vi "Test - Draw Teapot.vi"() -> ()   [LabVIEW 2022 SP3, in "Raster.lvlib"] (continued)
"y"=162.16495, "z"=0.9845819}, "UV"={"u"=0.0, "v"=0.0}, "Colour"=12517256}, "Vertex 2"={"Position"={"x"=543.45624, "y"=145.25499, "z"=0.98474205}, "UV"={"u"=0.0, "v"=0.0}, "Colour"=12517256}, "Vertex 3"={"Position"={"x"=502.52356, "y"=139.52065, "z"=0.9841747}, "UV"={"u"=0.0, "v"=0.0}, "Colour"=12517256}, "Alpha"=0.0, "Alpha Blending Enabled"=FALSE, "Colour"=5006902}, {"Vertex 1"={"Position"={"x"=354.40778, "y"=102.34398, "z"=0.9847698}, "UV"={"u"=0.0, "v"=0.0}, "Colour"=12517256}, "Vertex 2"={"Position"={"x"=351.39496, "y"=110.63302, "z"=0.984421}, "UV"={"u"=0.0, "v"=0.0}, "Colour"=12517256}, "Vertex 3"={"Position"={"x"=400.0, "y"=109.232285, "z"=0.9843054}, "UV"={"u"=0.0, "v"=0.0}, "Colour"=12517256}, "Alpha"=0.0, "Alpha Blending Enabled"=FALSE, "Colour"=395268}, {"Vertex 1"={"Position"={"x"=542.4723, "y"=251.44232, "z"=0.9847784}, "UV"={"u"=0.0, "v"=0.0}, "Colour"=12517256}, "Vertex 2"={"Position"={"x"=546.1793, "y"=227.81743, "z"=0.98464125}, "UV"={"u"=0.0, "v"=0.0}, "Colour"=12517256}, "Vertex 3"={"Position"={"x"=504.54324, "y"=225.08987, "z"=0.98405904}, "UV"={"u"=0.0, "v"=0.0}, "Colour"=12517256}, "Alpha"=0.0, "Alpha Blending Enabled"=FALSE, "Colour"=9947756}, {"Vertex 1"={"Position"={"x"=350.56738, "y"=298.80087, "z"=0.9843252}, "UV"={"u"=0.0, "v"=0.0}, "Colour"=12517256}, "Vertex 2"={"Position"={"x"=353.04034, "y"=323.3558, "z"=0.9846115}, "UV"={"u"=0.0, "v"=0.0}, "Colour"=12517256}, "Vertex 3"={"Position"={"x"=400.0, "y"=323.52267, "z"=0.9845012}, "UV"={"u"=0.0, "v"=0.0}, "Colour"=12517256}, "Alpha"=0.0, "Alpha Blending Enabled"=FALSE, "Colour"=11463036}, {"Vertex 1"={"Position"={"x"=301.7536, "y"=274.33585, "z"=0.9844198}, "UV"={"u"=0.0, "v"=0.0}, "Colour"=12517256}, "Vertex 2"={"Position"={"x"=298.20557, "y"=249.65573, "z"=0.9842166}, "UV"={"u"=0.0, "v"=0.0}, "Colour"=12517256}, "Vertex 3"={"Position"={"x"=257.52774, "y"=251.44232, "z"=0.9847784}, "UV"={"u"=0.0, "v"=0.0}, "Colour"=12517256}, "Alpha"=0.0, "Alpha Blending Enabled"=FALSE, "Colour"=10343024}, {"Vertex 1"={"Position"={"x"=301.7536, "y"=274.33585, "z"=0.9844198}, "UV"={"u"=0.0, "v"=0.0}, "Colour"=12517256}, "Vertex 2"={"Position"={"x"=305.9204, "y"=298.8263, "z"=0.9846586}, "UV"={"u"=0.0, "v"=0.0}, "Colour"=12517256}, "Vertex 3"={"Position"={"x"=350.56738, "y"=298.80087, "z"=0.9843252}, "UV"={"u"=0.0, "v"=0.0}, "Colour"=12517256}, "Alpha"=0.0, "Alpha Blending Enabled"=FALSE, "Colour"=11002232}, {"Vertex 1"={"Position"={"x"=400.0, "y"=100.973206, "z"=0.98466384}, "UV"={"u"=0.0, "v"=0.0}, "Colour"=12517256}, "Vertex 2"={"Position"={"x"=400.0, "y"=109.232285, "z"=0.9843054}, "UV"={"u"=0.0, "v"=0.0}, "Colour"=12517256}, "Vertex 3"={"Position"={"x"=448.60507, "y"=110.63302, "z"=0.984421}, "UV"={"u"=0.0, "v"=0.0}, "Colour"=12517256}, "Alpha"=0.0, "Alpha Blending Enabled"=FALSE, "Colour"=395268}, {"Vertex 1"={"Position"={"x"=497.92285, "y"=125.52894, "z"=0.98443836}, "UV"={"u"=0.0, "v"=0.0}, "Colour"=12517256}, "Vertex 2"={"Position"={"x"=502.52356, "y"=139.52065, "z"=0.9841747}, "UV"={"u"=0.0, "v"=0.0}, "Colour"=12517256}, "Vertex 3"={"Position"={"x"=543.45624, "y"=145.25499, "z"=0.98474205}, "UV"={"u"=0.0, "v"=0.0}, "Colour"=12517256}, "Alpha"=0.0, "Alpha Blending Enabled"=FALSE, "Colour"=2964512}, {"Vertex 1"={"Position"={"x"=400.0, "y"=298.79187, "z"=0.98420686}, "UV"={"u"=0.0, "v"=0.0}, "Colour"=12517256}, "Vertex 2"={"Position"={"x"=400.0, "y"=323.52267, "z"=0.9845012}, "UV"={"u"=0.0, "v"=0.0}, "Colour"=12517256}, "Vertex 3"={"Position"={"x"=446.95963, "y"=323.3558, "z"=0.9846115}, "UV"={"u"=0.0, "v"=0.0}, "Colour"=12517256}, "Alpha"=0.0, "Alpha Blending Enabled"=FALSE, "Colour"=11463036}, {"Vertex 1"={"Position"={"x"=256.5438, "y"=145.25499, "z"=0.98474205}, "UV"={"u"=0.0, "v"=0.0}, "Colour"=12517256}, "Vertex 2"={"Position"={"x"=252.2155, "y"=162.16495, "z"=0.9845819}, "UV"={"u"=0.0, "v"=0.0}, "Colour"=12517256}, "Vertex 3"={"Position"={"x"=294.26508, "y"=156.89722, "z"=0.9839907}, "UV"={"u"=0.0, "v"=0.0}, "Colour"=12517256}, "Alpha"=0.0, "Alpha Blending Enabled"=FALSE, "Colour"=5006902}, {"Vertex 1"={"Position"={"x"=307.46243, "y"=114.58211, "z"=0.98474693}, "UV"={"u"=0.0, "v"=0.0}, "Colour"=12517256}, "Vertex 2"={"Position"={"x"=302.07715, "y"=125.52894, "z"=0.98443836}, "UV"={"u"=0.0, "v"=0.0}, "Colour"=12517256}, "Vertex 3"={"Position"={"x"=348.50262, "y"=121.591866, "z"=0.98408604}, "UV"={"u"=0.0, "v"=0.0}, "Colour"=12517256}, "Alpha"=0.0, "Alpha Blending Enabled"=FALSE, "Colour"=1581073}, {"Vertex 1"={"Position"={"x"=348.50262, "y"=121.591866, "z"=0.98408604}, "UV"={"u"=0.0, "v"=0.0}, "Colour"=12517256}, "Vertex 2"={"Position"={"x"=351.39496, "y"=110.63302, "z"=0.984421}, "UV"={"u"=0.0, "v"=0.0}, "Colour"=12517256}, "Vertex 3"={"Position"={"x"=307.46243, "y"=114.58211, "z"=0.98474693}, "UV"={"u"=0.0, "v"=0.0}, "Colour"=12517256}, "Alpha"=0.0, "Alpha Blending Enabled"=FALSE, "Colour"=1581073}, {"Vertex 1"={"Position"={"x"=251.43709, "y"=204.66248, "z"=0.9845531}, "UV"={"u"=0.0, "v"=0.0}, "Colour"=12517256}, "Vertex 2"={"Position"={"x"=253.82066, "y"=227.81743, "z"=0.98464125}, "UV"={"u"=0.0, "v"=0.0}, "Colour"=12517256}, "Vertex 3"={"Position"={"x"=295.45676, "y"=225.08987, "z"=0.98405904}, "UV"={"u"=0.0, "v"=0.0}, "Colour"=12517256}, "Alpha"=0.0, "Alpha Blending Enabled"=FALSE, "Colour"=9355110}, {"Vertex 1"={"Position"={"x"=546.1793, "y"=227.81743, "z"=0.98464125}, "UV"={"u"=0.0, "v"=0.0}, "Colour"=12517256}, "Vertex 2"={"Position"={"x"=548.5629, "y"=204.66248, "z"=0.9845531}, "UV"={"u"=0.0, "v"=0.0}, "Colour"=12517256}, "Vertex 3"={"Position"={"x"=506.31323, "y"=200.99902, "z"=0.98395765}, "UV"={"u"=0.0, "v"=0.0}, "Colour"=12517256}, "Alpha"=0.0, "Alpha Blending Enabled"=FALSE, "Colour"=9355110}, {"Vertex 1"={"Position"={"x"=494.0796, "y"=298.8263, "z"=0.9846586}, "UV"={"u"=0.0, "v"=0.0}, "Colour"=12517256}, "Vertex 2"={"Position"={"x"=498.2464, "y"=274.33585, "z"=0.9844198}, "UV"={"u"=0.0, "v"=0.0}, "Colour"=12517256}, "Vertex 3"={"Position"={"x"=451.6715, "y"=273.75476, "z"=0.9840659}, "UV"={"u"=0.0, "v"=0.0}, "Colour"=12517256}, "Alpha"=0.0, "Alpha Blending Enabled"=FALSE, "Colour"=11002232}, {"Vertex 1"={"Position"={"x"=446.95963, "y"=323.3558, "z"=0.9846115}, "UV"={"u"=0.0, "v"=0.0}, "Colour"=12517256}, "Vertex 2"={"Position"={"x"=449.43246, "y"=298.80087, "z"=0.9843252}, "UV"={"u"=0.0, "v"=0.0}, "Colour"=12517256}, "Vertex 3"={"Position"={"x"=400.0, "y"=298.79187, "z"=0.98420686}, "UV"={"u"=0.0, "v"=0.0}, "Colour"=12517256}, "Alpha"=0.0, "Alpha Blending Enabled"=FALSE, "Colour"=11463036}, {"Vertex 1"={"Position"={"x"=549.402, "y"=182.33759, "z"=0.9845221}, "UV"={"u"=0.0, "v"=0.0}, "Colour"=12517256}, "Vertex 2"={"Position"={"x"=547.78455, "y"=162.16495, "z"=0.9845819}, "UV"={"u"=0.0, "v"=0.0}, "Colour"=12517256}, "Vertex 3"={"Position"={"x"=505.73492, "y"=156.89722, "z"=0.9839907}, "UV"={"u"=0.0, "v"=0.0}, "Colour"=12517256}, "Alpha"=0.0, "Alpha Blending Enabled"=FALSE, "Colour"=7180878}, {"Vertex 1"={"Position"={"x"=504.54324, "y"=225.08987, "z"=0.98405904}, "UV"={"u"=0.0, "v"=0.0}, "Colour"=12517256}, "Vertex 2"={"Position"={"x"=501.79443, "y"=249.65573, "z"=0.9842166}, "UV"={"u"=0.0, "v"=0.0}, "Colour"=12517256}, "Vertex 3"={"Position"={"x"=542.4723, "y"=251.44232, "z"=0.9847784}, "UV"={"u"=0.0, "v"=0.0}, "Colour"=12517256}, "Alpha"=0.0, "Alpha Blending Enabled"=FALSE, "Colour"=9947756}, {"Vertex 1"={"Position"={"x"=451.6715, "y"=273.75476, "z"=0.9840659}, "UV"={"u"=0.0, "v"=0.0}, "Colour"=12517256}, "Vertex 2"={"Position"={"x"=449.43246, "y"=298.80087, "z"=0.9843252}, "UV"={"u"=0.0, "v"=0.0}, "Colour"=12517256}, "Vertex 3"={"Position"={"x"=494.0796, "y"=298.8263, "z"=0.9846586}, "UV"={"u"=0.0, "v"=0.0}, "Colour"=12517256}, "Alpha"=0.0, "Alpha Blending Enabled"=FALSE, "Colour"=11002232}, {"Vertex 1"={"Position"={"x"=400.0, "y"=323.52267, "z"=0.9845012}, "UV"={"u"=0.0, "v"=0.0}, "Colour"=12517256}, "Vertex 2"={"Position"={"x"=400.0, "y"=298.79187, "z"=0.98420686}, "UV"={"u"=0.0, "v"=0.0}, "Colour"=12517256}, "Vertex 3"={"Position"={"x"=350.56738, "y"=298.80087, "z"=0.9843252}, "UV"={"u"=0.0, "v"=0.0}, "Colour"=12517256}, "Alpha"=0.0, "Alpha Blending Enabled"=FALSE, "Colour"=11463036}, {"Vertex 1"={"Position"={"x"=250.598, "y"=182.33759, "z"=0.9845221}, "UV"={"u"=0.0, "v"=0.0}, "Colour"=12517256}, "Vertex 2"={"Position"={"x"=251.43709, "y"=204.66248, "z"=0.9845531}, "UV"={"u"=0.0, "v"=0.0}, "Colour"=12517256}, "Vertex 3"={"Position"={"x"=293.68674, "y"=200.99902, "z"=0.98395765}, "UV"={"u"=0.0, "v"=0.0}, "Colour"=12517256}, "Alpha"=0.0, "Alpha Blending Enabled"=FALSE, "Colour"=8630366}, {"Vertex 1"={"Position"={"x"=252.2155, "y"=162.16495, "z"=0.9845819}, "UV"={"u"=0.0, "v"=0.0}, "Colour"=12517256}, "Vertex 2"={"Position"={"x"=250.598, "y"=182.33759, "z"=0.9845221}, "UV"={"u"=0.0, "v"=0.0}, "Colour"=12517256}, "Vertex 3"={"Position"={"x"=293.06296, "y"=177.78967, "z"=0.9839219}, "UV"={"u"=0.0, "v"=0.0}, "Colour"=12517256}, "Alpha"=0.0, "Alpha Blending Enabled"=FALSE, "Colour"=7180878}, {"Vertex 1"={"Position"={"x"=548.5629, "y"=204.66248, "z"=0.9845531}, "UV"={"u"=0.0, "v"=0.0}, "Colour"=12517256}, "Vertex 2"={"Position"={"x"=549.402, "y"=182.33759, "z"=0.9845221}, "UV"={"u"=0.0, "v"=0.0}, "Colour"=12517256}, "Vertex 3"={"Position"={"x"=506.937, "y"=177.78967, "z"=0.9839219}, "UV"={"u"=0.0, "v"=0.0}, "Colour"=12517256}, "Alpha"=0.0, "Alpha Blending Enabled"=FALSE, "Colour"=8630366}, {"Vertex 1"={"Position"={"x"=448.60507, "y"=110.63302, "z"=0.984421}, "UV"={"u"=0.0, "v"=0.0}, "Colour"=12517256}, "Vertex 2"={"Position"={"x"=451.49738, "y"=121.591866, "z"=0.98408604}, "UV"={"u"=0.0, "v"=0.0}, "Colour"=12517256}, "Vertex 3"={"Position"={"x"=497.92285, "y"=125.52894, "z"=0.98443836}, "UV"={"u"=0.0, "v"=0.0}, "Colour"=12517256}, "Alpha"=0.0, "Alpha Blending Enabled"=FALSE, "Colour"=1581073}, {"Vertex 1"={"Position"={"x"=298.20557, "y"=249.65573, "z"=0.9842166}, "UV"={"u"=0.0, "v"=0.0}, "Colour"=12517256}, "Vertex 2"={"Position"={"x"=295.45676, "y"=225.08987, "z"=0.98405904}, "UV"={"u"=0.0, "v"=0.0}, "Colour"=12517256}, "Vertex 3"={"Position"={"x"=253.82066, "y"=227.81743, "z"=0.98464125}, "UV"={"u"=0.0, "v"=0.0}, "Colour"=12517256}, "Alpha"=0.0, "Alpha Blending Enabled"=FALSE, "Colour"=9947756}, {"Vertex 1"={"Position"={"x"=294.26508, "y"=156.89722, "z"=0.9839907}, "UV"={"u"=0.0, "v"=0.0}, "Colour"=12517256}, "Vertex 2"={"Position"={"x"=297.47644, "y"=139.52065, "z"=0.9841747}, "UV"={"u"=0.0, "v"=0.0}, "Colour"=12517256}, "Vertex 3"={"Position"={"x"=256.5438, "y"=145.25499, "z"=0.98474205}, "UV"={"u"=0.0, "v"=0.0}, "Colour"=12517256}, "Alpha"=0.0, "Alpha Blending Enabled"=FALSE, "Colour"=5006902}, {"Vertex 1"={"Position"={"x"=451.49738, "y"=121.591866, "z"=0.98408604}, "UV"={"u"=0.0, "v"=0.0}, "Colour"=12517256}, "Vertex 2"={"Position"={"x"=448.60507, "y"=110.63302, "z"=0.984421}, "UV"={"u"=0.0, "v"=0.0}, "Colour"=12517256}, "Vertex 3"={"Position"={"x"=400.0, "y"=109.232285, "z"=0.9843054}, "UV"={"u"=0.0, "v"=0.0}, "Colour"=12517256}, "Alpha"=0.0, "Alpha Blending Enabled"=FALSE, "Colour"=1778707}, {"Vertex 1"={"Position"={"x"=350.56738, "y"=298.80087, "z"=0.9843252}, "UV"={"u"=0.0, "v"=0.0}, "Colour"=12517256}, "Vertex 2"={"Position"={"x"=348.32846, "y"=273.75476, "z"=0.9840659}, "UV"={"u"=0.0, "v"=0.0}, "Colour"=12517256}, "Vertex 3"={"Position"={"x"=301.7536, "y"=274.33585, "z"=0.9844198}, "UV"={"u"=0.0, "v"=0.0}, "Colour"=12517256}, "Alpha"=0.0, "Alpha Blending Enabled"=FALSE, "Colour"=11002232}, {"Vertex 1"={"Position"={"x"=502.52356, "y"=139.52065, "z"=0.9841747}, "UV"={"u"=0.0, "v"=0.0}, "Colour"=12517256}, "Vertex 2"={"Position"={"x"=505.73492, "y"=156.89722, "z"=0.9839907}, "UV"={"u"=0.0, "v"=0.0}, "Colour"=12517256}, "Vertex 3"={"Position"={"x"=547.78455, "y"=162.16495, "z"=0.9845819}, "UV"={"u"=0.0, "v"=0.0}, "Colour"=12517256}, "Alpha"=0.0, "Alpha Blending Enabled"=FALSE, "Colour"=5006902}, {"Vertex 1"={"Position"={"x"=298.20557, "y"=249.65573, "z"=0.9842166}, "UV"={"u"=0.0, "v"=0.0}, "Colour"=12517256}, "Vertex 2"={"Position"={"x"=301.7536, "y"=274.33585, "z"=0.9844198}, "UV"={"u"=0.0, "v"=0.0}, "Colour"=12517256}, "Vertex 3"={"Position"={"x"=348.32846, "y"=273.75476, "z"=0.9840659}, "UV"={"u"=0.0, "v"=0.0}, "Colour"=12517256}, "Alpha"=0.0, "Alpha Blending Enabled"=FALSE, "Colour"=10738549}, {"Vertex 1"={"Position"={"x"=502.52356, "y"=139.52065, "z"=0.9841747}, "UV"={"u"=0.0, "v"=0.0}, "Colour"=12517256}, "Vertex 2"={"Position"={"x"=497.92285, "y"=125.52894, "z"=0.98443836}, "UV"={"u"=0.0, "v"=0.0}, "Colour"=12517256}, "Vertex 3"={"Position"={"x"=451.49738, "y"=121.591866, "z"=0.98408604}, "UV"={"u"=0.0, "v"=0.0}, "Colour"=12517256}, "Alpha"=0.0, "Alpha Blending Enabled"=FALSE, "Colour"=3294244}, {"Vertex 1"={"Position"={"x"=400.0, "y"=120.19295, "z"=0.98396087}, "UV"={"u"=0.0, "v"=0.0}, "Colour"=12517256}, "Vertex 2"={"Position"={"x"=400.0, "y"=109.232285, "z"=0.9843054}, "UV"={"u"=0.0, "v"=0.0}, "Colour"=12517256}, "Vertex 3"={"Position"={"x"=351.39496, "y"=110.63302, "z"=0.984421}, "UV"={"u"=0.0, "v"=0.0}, "Colour"=12517256}, "Alpha"=0.0, "Alpha Blending Enabled"=FALSE, "Colour"=1778707}, {"Vertex 1"={"Position"={"x"=506.31323, "y"=200.99902, "z"=0.98395765}, "UV"={"u"=0.0, "v"=0.0}, "Colour"=12517256}, "Vertex 2"={"Position"={"x"=504.54324, "y"=225.08987, "z"=0.98405904}, "UV"={"u"=0.0, "v"=0.0}, "Colour"=12517256}, "Vertex 3"={"Position"={"x"=546.1793, "y"=227.81743, "z"=0.98464125}, "UV"={"u"=0.0, "v"=0.0}, "Colour"=12517256}, "Alpha"=0.0, "Alpha Blending Enabled"=FALSE, "Colour"=9355110}, {"Vertex 1"={"Position"={"x"=348.32846, "y"=273.75476, "z"=0.9840659}, "UV"={"u"=0.0, "v"=0.0}, "Colour"=12517256}, "Vertex 2"={"Position"={"x"=350.56738, "y"=298.80087, "z"=0.9843252}, "UV"={"u"=0.0, "v"=0.0}, "Colour"=12517256}, "Vertex 3"={"Position"={"x"=400.0, "y"=298.79187, "z"=0.98420686}, "UV"={"u"=0.0, "v"=0.0}, "Colour"=12517256}, "Alpha"=0.0, "Alpha Blending Enabled"=FALSE, "Colour"=11199866}, {"Vertex 1"={"Position"={"x"=295.45676, "y"=225.08987, "z"=0.98405904}, "UV"={"u"=0.0, "v"=0.0}, "Colour"=12517256}, "Vertex 2"={"Position"={"x"=293.68674, "y"=200.99902, "z"=0.98395765}, "UV"={"u"=0.0, "v"=0.0}, "Colour"=12517256}, "Vertex 3"={"Position"={"x"=251.43709, "y"=204.66248, "z"=0.9845531}, "UV"={"u"=0.0, "v"=0.0}, "Colour"=12517256}, "Alpha"=0.0, "Alpha Blending Enabled"=FALSE, "Colour"=9355110}, {"Vertex 1"={"Position"={"x"=293.06296, "y"=177.78967, "z"=0.9839219}, "UV"={"u"=0.0, "v"=0.0}, "Colour"=12517256}, "Vertex 2"={"Position"={"x"=294.26508, "y"=156.89722, "z"=0.9839907}, "UV"={"u"=0.0, "v"=0.0}, "Colour"=12517256}, "Vertex 3"={"Position"={"x"=252.2155, "y"=162.16495, "z"=0.9845819}, "UV"={"u"=0.0, "v"=0.0}, "Colour"=12517256}, "Alpha"=0.0, "Alpha Blending Enabled"=FALSE, "Colour"=7180878}, {"Vertex 1"={"Position"={"x"=498.2464, "y"=274.33585, "z"=0.9844198}, "UV"={"u"=0.0, "v"=0.0}, "Colour"=12517256}, "Vertex 2"={"Position"={"x"=501.79443, "y"=249.65573, "z"=0.9842166}, "UV"={"u"=0.0, "v"=0.0}, "Colour"=12517256}, "Vertex 3"={"Position"={"x"=453.58133, "y"=248.47368, "z"=0.98384476}, "UV"={"u"=0.0, "v"=0.0}, "Colour"=12517256}, "Alpha"=0.0, "Alpha Blending Enabled"=FALSE, "Colour"=10738549}, {"Vertex 1"={"Position"={"x"=400.0, "y"=273.54828, "z"=0.9839401}, "UV"={"u"=0.0, "v"=0.0}, "Colour"=12517256}, "Vertex 2"={"Position"={"x"=400.0, "y"=298.79187, "z"=0.98420686}, "UV"={"u"=0.0, "v"=0.0}, "Colour"=12517256}, "Vertex 3"={"Position"={"x"=449.43246, "y"=298.80087, "z"=0.9843252}, "UV"={"u"=0.0, "v"=0.0}, "Colour"=12517256}, "Alpha"=0.0, "Alpha Blending Enabled"=FALSE, "Colour"=11199866}, {"Vertex 1"={"Position"={"x"=351.39496, "y"=110.63302, "z"=0.984421}, "UV"={"u"=0.0, "v"=0.0}, "Colour"=12517256}, "Vertex 2"={"Position"={"x"=348.50262, "y"=121.591866, "z"=0.98408604}, "UV"={"u"=0.0, "v"=0.0}, "Colour"=12517256}, "Vertex 3"={"Position"={"x"=400.0, "y"=120.19295, "z"=0.98396087}, "UV"={"u"=0.0, "v"=0.0}, "Colour"=12517256}, "Alpha"=0.0, "Alpha Blending Enabled"=FALSE, "Colour"=1778707}, {"Vertex 1"={"Position"={"x"=505.73492, "y"=156.89722, "z"=0.9839907}, "UV"={"u"=0.0, "v"=0.0}, "Colour"=12517256}, "Vertex 2"={"Position"={"x"=506.937, "y"=177.78967, "z"=0.9839219}, "UV"={"u"=0.0, "v"=0.0}, "Colour"=12517256}, "Vertex 3"={"Position"={"x"=549.402, "y"=182.33759, "z"=0.9845221}, "UV"={"u"=0.0, "v"=0.0}, "Colour"=12517256}, "Alpha"=0.0, "Alpha Blending Enabled"=FALSE, "Colour"=7180878}, {"Vertex 1"={"Position"={"x"=506.937, "y"=177.78967, "z"=0.9839219}, "UV"={"u"=0.0, "v"=0.0}, "Colour"=12517256}, "Vertex 2"={"Position"={"x"=506.31323, "y"=200.99902, "z"=0.98395765}, "UV"={"u"=0.0, "v"=0.0}, "Colour"=12517256}, "Vertex 3"={"Position"={"x"=548.5629, "y"=204.66248, "z"=0.9845531}, "UV"={"u"=0.0, "v"=0.0}, "Colour"=12517256}, "Alpha"=0.0, "Alpha Blending Enabled"=FALSE, "Colour"=8630366}, {"Vertex 1"={"Position"={"x"=302.07715, "y"=125.52894, "z"=0.98443836}, "UV"={"u"=0.0, "v"=0.0}, "Colour"=12517256}, "Vertex 2"={"Position"={"x"=297.47644, "y"=139.52065, "z"=0.9841747}, "UV"={"u"=0.0, "v"=0.0}, "Colour"=12517256}, "Vertex 3"={"Position"={"x"=346.02576, "y"=135.72502, "z"=0.9837993}, "UV"={"u"=0.0, "v"=0.0}, "Colour"=12517256}, "Alpha"=0.0, "Alpha Blending Enabled"=FALSE, "Colour"=3294244}, {"Vertex 1"={"Position"={"x"=293.68674, "y"=200.99902, "z"=0.98395765}, "UV"={"u"=0.0, "v"=0.0}, "Colour"=12517256}, "Vertex 2"={"Position"={"x"=293.06296, "y"=177.78967, "z"=0.9839219}, "UV"={"u"=0.0, "v"=0.0}, "Colour"=12517256}, "Vertex 3"={"Position"={"x"=250.598, "y"=182.33759, "z"=0.9845221}, "UV"={"u"=0.0, "v"=0.0}, "Colour"=12517256}, "Alpha"=0.0, "Alpha Blending Enabled"=FALSE, "Colour"=8630366}, {"Vertex 1"={"Position"={"x"=400.0, "y"=109.232285, "z"=0.9843054}, "UV"={"u"=0.0, "v"=0.0}, "Colour"=12517256}, "Vertex 2"={"Position"={"x"=400.0, "y"=120.19295, "z"=0.98396087}, "UV"={"u"=0.0, "v"=0.0}, "Colour"=12517256}, "Vertex 3"={"Position"={"x"=451.49738, "y"=121.591866, "z"=0.98408604}, "UV"={"u"=0.0, "v"=0.0}, "Colour"=12517256}, "Alpha"=0.0, "Alpha Blending Enabled"=FALSE, "Colour"=1778707}, {"Vertex 1"={"Position"={"x"=449.43246, "y"=298.80087, "z"=0.9843252}, "UV"={"u"=0.0, "v"=0.0}, "Colour"=12517256}, "Vertex 2"={"Position"={"x"=451.6715, "y"=273.75476, "z"=0.9840659}, "UV"={"u"=0.0, "v"=0.0}, "Colour"=12517256}, "Vertex 3"={"Position"={"x"=400.0, "y"=273.54828, "z"=0.9839401}, "UV"={"u"=0.0, "v"=0.0}, "Colour"=12517256}, "Alpha"=0.0, "Alpha Blending Enabled"=FALSE, "Colour"=11199866}, {"Vertex 1"={"Position"={"x"=453.58133, "y"=248.47368, "z"=0.98384476}, "UV"={"u"=0.0, "v"=0.0}, "Colour"=12517256}, "Vertex 2"={"Position"={"x"=451.6715, "y"=273.75476, "z"=0.9840659}, "UV"={"u"=0.0, "v"=0.0}, "Colour"=12517256}, "Vertex 3"={"Position"={"x"=498.2464, "y"=274.33585, "z"=0.9844198}, "UV"={"u"=0.0, "v"=0.0}, "Colour"=12517256}, "Alpha"=0.0, "Alpha Blending Enabled"=FALSE, "Colour"=10738549}, {"Vertex 1"={"Position"={"x"=346.02576, "y"=135.72502, "z"=0.9837993}, "UV"={"u"=0.0, "v"=0.0}, "Colour"=12517256}, "Vertex 2"={"Position"={"x"=348.50262, "y"=121.591866, "z"=0.98408604}, "UV"={"u"=0.0, "v"=0.0}, "Colour"=12517256}, "Vertex 3"={"Position"={"x"=302.07715, "y"=125.52894, "z"=0.98443836}, "UV"={"u"=0.0, "v"=0.0}, "Colour"=12517256}, "Alpha"=0.0, "Alpha Blending Enabled"=FALSE, "Colour"=3294244}, {"Vertex 1"={"Position"={"x"=400.0, "y"=298.79187, "z"=0.98420686}, "UV"={"u"=0.0, "v"=0.0}, "Colour"=12517256}, "Vertex 2"={"Position"={"x"=400.0, "y"=273.54828, "z"=0.9839401}, "UV"={"u"=0.0, "v"=0.0}, "Colour"=12517256}, "Vertex 3"={"Position"={"x"=348.32846, "y"=273.75476, "z"=0.9840659}, "UV"={"u"=0.0, "v"=0.0}, "Colour"=12517256}, "Alpha"=0.0, "Alpha Blending Enabled"=FALSE, "Colour"=11199866}, {"Vertex 1"={"Position"={"x"=348.32846, "y"=273.75476, "z"=0.9840659}, "UV"={"u"=0.0, "v"=0.0}, "Colour"=12517256}, "Vertex 2"={"Position"={"x"=346.41867, "y"=248.47368, "z"=0.98384476}, "UV"={"u"=0.0, "v"=0.0}, "Colour"=12517256}, "Vertex 3"={"Position"={"x"=298.20557, "y"=249.65573, "z"=0.9842166}, "UV"={"u"=0.0, "v"=0.0}, "Colour"=12517256}, "Alpha"=0.0, "Alpha Blending Enabled"=FALSE, "Colour"=10738549}, {"Vertex 1"={"Position"={"x"=295.45676, "y"=225.08987, "z"=0.98405904}, "UV"={"u"=0.0, "v"=0.0}, "Colour"=12517256}, "Vertex 2"={"Position"={"x"=298.20557, "y"=249.65573, "z"=0.9842166}, "UV"={"u"=0.0, "v"=0.0}, "Colour"=12517256}, "Vertex 3"={"Position"={"x"=346.41867, "y"=248.47368, "z"=0.98384476}, "UV"={"u"=0.0, "v"=0.0}, "Colour"=12517256}, "Alpha"=0.0, "Alpha Blending Enabled"=FALSE, "Colour"=10343280}, {"Vertex 1"={"Position"={"x"=451.49738, "y"=121.591866, "z"=0.98408604}, "UV"={"u"=0.0, "v"=0.0}, "Colour"=12517256}, "Vertex 2"={"Position"={"x"=453.97424, "y"=135.72502, "z"=0.9837993}, "UV"={"u"=0.0, "v"=0.0}, "Colour"=12517256}, "Vertex 3"={"Position"={"x"=502.52356, "y"=139.52065, "z"=0.9841747}, "UV"={"u"=0.0, "v"=0.0}, "Colour"=12517256}, "Alpha"=0.0, "Alpha Blending Enabled"=FALSE, "Colour"=3294244}, {"Vertex 1"={"Position"={"x"=505.73492, "y"=156.89722, "z"=0.9839907}, "UV"={"u"=0.0, "v"=0.0}, "Colour"=12517256}, "Vertex 2"={"Position"={"x"=502.52356, "y"=139.52065, "z"=0.9841747}, "UV"={"u"=0.0, "v"=0.0}, "Colour"=12517256}, "Vertex 3"={"Position"={"x"=453.97424, "y"=135.72502, "z"=0.9837993}, "UV"={"u"=0.0, "v"=0.0}, "Colour"=12517256}, "Alpha"=0.0, "Alpha Blending Enabled"=FALSE, "Colour"=5402171}, {"Vertex 1"={"Position"={"x"=501.79443, "y"=249.65573, "z"=0.9842166}, "UV"={"u"=0.0, "v"=0.0}, "Colour"=12517256}, "Vertex 2"={"Position"={"x"=504.54324, "y"=225.08987, "z"=0.98405904}, "UV"={"u"=0.0, "v"=0.0}, "Colour"=12517256}, "Vertex 3"={"Position"={"x"=455.0632, "y"=223.28236, "z"=0.9836732}, "UV"={"u"=0.0, "v"=0.0}, "Colour"=12517256}, "Alpha"=0.0, "Alpha Blending Enabled"=FALSE, "Colour"=10343280}, {"Vertex 1"={"Position"={"x"=346.41867, "y"=248.47368, "z"=0.98384476}, "UV"={"u"=0.0, "v"=0.0}, "Colour"=12517256}, "Vertex 2"={"Position"={"x"=348.32846, "y"=273.75476, "z"=0.9840659}, "UV"={"u"=0.0, "v"=0.0}, "Colour"=12517256}, "Vertex 3"={"Position"={"x"=400.0, "y"=273.54828, "z"=0.9839401}, "UV"={"u"=0.0, "v"=0.0}, "Colour"=12517256}, "Alpha"=0.0, "Alpha Blending Enabled"=FALSE, "Colour"=10936183}, {"Vertex 1"={"Position"={"x"=453.97424, "y"=135.72502, "z"=0.9837993}, "UV"={"u"=0.0, "v"=0.0}, "Colour"=12517256}, "Vertex 2"={"Position"={"x"=451.49738, "y"=121.591866, "z"=0.98408604}, "UV"={"u"=0.0, "v"=0.0}, "Colour"=12517256}, "Vertex 3"={"Position"={"x"=400.0, "y"=120.19295, "z"=0.98396087}, "UV"={"u"=0.0, "v"=0.0}, "Colour"=12517256}, "Alpha"=0.0, "Alpha Blending Enabled"=FALSE, "Colour"=3491878}, {"Vertex 1"={"Position"={"x"=297.47644, "y"=139.52065, "z"=0.9841747}, "UV"={"u"=0.0, "v"=0.0}, "Colour"=12517256}, "Vertex 2"={"Position"={"x"=294.26508, "y"=156.89722, "z"=0.9839907}, "UV"={"u"=0.0, "v"=0.0}, "Colour"=12517256}, "Vertex 3"={"Position"={"x"=344.29382, "y"=153.40399, "z"=0.9835987}, "UV"={"u"=0.0, "v"=0.0}, "Colour"=12517256}, "Alpha"=0.0, "Alpha Blending Enabled"=FALSE, "Colour"=5402171}, {"Vertex 1"={"Position"={"x"=455.0632, "y"=223.28236, "z"=0.9836732}, "UV"={"u"=0.0, "v"=0.0}, "Colour"=12517256}, "Vertex 2"={"Position"={"x"=453.58133, "y"=248.47368, "z"=0.98384476}, "UV"={"u"=0.0, "v"=0.0}, "Colour"=12517256}, "Vertex 3"={"Position"={"x"=501.79443, "y"=249.65573, "z"=0.9842166}, "UV"={"u"=0.0, "v"=0.0}, "Colour"=12517256}, "Alpha"=0.0, "Alpha Blending Enabled"=FALSE, "Colour"=10343280}, {"Vertex 1"={"Position"={"x"=400.0, "y"=248.05318, "z"=0.98371255}, "UV"={"u"=0.0, "v"=0.0}, "Colour"=12517256}, "Vertex 2"={"Position"={"x"=400.0, "y"=273.54828, "z"=0.9839401}, "UV"={"u"=0.0, "v"=0.0}, "Colour"=12517256}, "Vertex 3"={"Position"={"x"=451.6715, "y"=273.75476, "z"=0.9840659}, "UV"={"u"=0.0, "v"=0.0}, "Colour"=12517256}, "Alpha"=0.0, "Alpha Blending Enabled"=FALSE, "Colour"=10936183}, {"Vertex 1"={"Position"={"x"=400.0, "y"=134.37457, "z"=0.9836657}, "UV"={"u"=0.0, "v"=0.0}, "Colour"=12517256}, "Vertex 2"={"Position"={"x"=400.0, "y"=120.19295, "z"=0.98396087}, "UV"={"u"=0.0, "v"=0.0}, "Colour"=12517256}, "Vertex 3"={"Position"={"x"=348.50262, "y"=121.591866, "z"=0.98408604}, "UV"={"u"=0.0, "v"=0.0}, "Colour"=12517256}, "Alpha"=0.0, "Alpha Blending Enabled"=FALSE, "Colour"=3491878}, {"Vertex 1"={"Position"={"x"=293.68674, "y"=200.99902, "z"=0.98395765}, "UV"={"u"=0.0, "v"=0.0}, "Colour"=12517256}, "Vertex 2"={"Position"={"x"=295.45676, "y"=225.08987, "z"=0.98405904}, "UV"={"u"=0.0, "v"=0.0}, "Colour"=12517256}, "Vertex 3"={"Position"={"x"=344.93683, "y"=223.28236, "z"=0.9836732}, "UV"={"u"=0.0, "v"=0.0}, "Colour"=12517256}, "Alpha"=0.0, "Alpha Blending Enabled"=FALSE, "Colour"=9816170}, {"Vertex 1"={"Position"={"x"=451.6715, "y"=273.75476, "z"=0.9840659}, "UV"={"u"=0.0, "v"=0.0}, "Colour"=12517256}, "Vertex 2"={"Position"={"x"=453.58133, "y"=248.47368, "z"=0.98384476}, "UV"={"u"=0.0, "v"=0.0}, "Colour"=12517256}, "Vertex 3"={"Position"={"x"=400.0, "y"=248.05318, "z"=0.98371255}, "UV"={"u"=0.0, "v"=0.0}, "Colour"=12517256}, "Alpha"=0.0, "Alpha Blending Enabled"=FALSE, "Colour"=10936183}, {"Vertex 1"={"Position"={"x"=504.54324, "y"=225.08987, "z"=0.98405904}, "UV"={"u"=0.0, "v"=0.0}, "Colour"=12517256}, "Vertex 2"={"Position"={"x"=506.31323, "y"=200.99902, "z"=0.98395765}, "UV"={"u"=0.0, "v"=0.0}, "Colour"=12517256}, "Vertex 3"={"Position"={"x"=456.01822, "y"=198.56883, "z"=0.9835626}, "UV"={"u"=0.0, "v"=0.0}, "Colour"=12517256}, "Alpha"=0.0, "Alpha Blending Enabled"=FALSE, "Colour"=9816170}, {"Vertex 1"={"Position"={"x"=346.41867, "y"=248.47368, "z"=0.98384476}, "UV"={"u"=0.0, "v"=0.0}, "Colour"=12517256}, "Vertex 2"={"Position"={"x"=344.93683, "y"=223.28236, "z"=0.9836732}, "UV"={"u"=0.0, "v"=0.0}, "Colour"=12517256}, "Vertex 3"={"Position"={"x"=295.45676, "y"=225.08987, "z"=0.98405904}, "UV"={"u"=0.0, "v"=0.0}, "Colour"=12517256}, "Alpha"=0.0, "Alpha Blending Enabled"=FALSE, "Colour"=10343280}, {"Vertex 1"={"Position"={"x"=344.29382, "y"=153.40399, "z"=0.9835987}, "UV"={"u"=0.0, "v"=0.0}, "Colour"=12517256}, "Vertex 2"={"Position"={"x"=346.02576, "y"=135.72502, "z"=0.9837993}, "UV"={"u"=0.0, "v"=0.0}, "Colour"=12517256}, "Vertex 3"={"Position"={"x"=297.47644, "y"=139.52065, "z"=0.9841747}, "UV"={"u"=0.0, "v"=0.0}, "Colour"=12517256}, "Alpha"=0.0, "Alpha Blending Enabled"=FALSE, "Colour"=5402171}, {"Vertex 1"={"Position"={"x"=348.50262, "y"=121.591866, "z"=0.98408604}, "UV"={"u"=0.0, "v"=0.0}, "Colour"=12517256}, "Vertex 2"={"Position"={"x"=346.02576, "y"=135.72502, "z"=0.9837993}, "UV"={"u"=0.0, "v"=0.0}, "Colour"=12517256}, "Vertex 3"={"Position"={"x"=400.0, "y"=134.37457, "z"=0.9836657}, "UV"={"u"=0.0, "v"=0.0}, "Colour"=12517256}, "Alpha"=0.0, "Alpha Blending Enabled"=FALSE, "Colour"=3491878}, {"Vertex 1"={"Position"={"x"=506.937, "y"=177.78967, "z"=0.9839219}, "UV"={"u"=0.0, "v"=0.0}, "Colour"=12517256}, "Vertex 2"={"Position"={"x"=505.73492, "y"=156.89722, "z"=0.9839907}, "UV"={"u"=0.0, "v"=0.0}, "Colour"=12517256}, "Vertex 3"={"Position"={"x"=455.7062, "y"=153.40399, "z"=0.9835987}, "UV"={"u"=0.0, "v"=0.0}, "Colour"=12517256}, "Alpha"=0.0, "Alpha Blending Enabled"=FALSE, "Colour"=7576403}, {"Vertex 1"={"Position"={"x"=400.0, "y"=273.54828, "z"=0.9839401}, "UV"={"u"=0.0, "v"=0.0}, "Colour"=12517256}, "Vertex 2"={"Position"={"x"=400.0, "y"=248.05318, "z"=0.98371255}, "UV"={"u"=0.0, "v"=0.0}, "Colour"=12517256}, "Vertex 3"={"Position"={"x"=346.41867, "y"=248.47368, "z"=0.98384476}, "UV"={"u"=0.0, "v"=0.0}, "Colour"=12517256}, "Alpha"=0.0, "Alpha Blending Enabled"=FALSE, "Colour"=10936183}, {"Vertex 1"={"Position"={"x"=293.06296, "y"=177.78967, "z"=0.9839219}, "UV"={"u"=0.0, "v"=0.0}, "Colour"=12517256}, "Vertex 2"={"Position"={"x"=293.68674, "y"=200.99902, "z"=0.98395765}, "UV"={"u"=0.0, "v"=0.0}, "Colour"=12517256}, "Vertex 3"={"Position"={"x"=343.98178, "y"=198.56883, "z"=0.9835626}, "UV"={"u"=0.0, "v"=0.0}, "Colour"=12517256}, "Alpha"=0.0, "Alpha Blending Enabled"=FALSE, "Colour"=9091426}, {"Vertex 1"={"Position"={"x"=294.26508, "y"=156.89722, "z"=0.9839907}, "UV"={"u"=0.0, "v"=0.0}, "Colour"=12517256}, "Vertex 2"={"Position"={"x"=293.06296, "y"=177.78967, "z"=0.9839219}, "UV"={"u"=0.0, "v"=0.0}, "Colour"=12517256}, "Vertex 3"={"Position"={"x"=343.64493, "y"=174.77179, "z"=0.9835236}, "UV"={"u"=0.0, "v"=0.0}, "Colour"=12517256}, "Alpha"=0.0, "Alpha Blending Enabled"=FALSE, "Colour"=7576403}, {"Vertex 1"={"Position"={"x"=400.0, "y"=120.19295, "z"=0.98396087}, "UV"={"u"=0.0, "v"=0.0}, "Colour"=12517256}, "Vertex 2"={"Position"={"x"=400.0, "y"=134.37457, "z"=0.9836657}, "UV"={"u"=0.0, "v"=0.0}, "Colour"=12517256}, "Vertex 3"={"Position"={"x"=453.97424, "y"=135.72502, "z"=0.9837993}, "UV"={"u"=0.0, "v"=0.0}, "Colour"=12517256}, "Alpha"=0.0, "Alpha Blending Enabled"=FALSE, "Colour"=3491878}, {"Vertex 1"={"Position"={"x"=506.31323, "y"=200.99902, "z"=0.98395765}, "UV"={"u"=0.0, "v"=0.0}, "Colour"=12517256}, "Vertex 2"={"Position"={"x"=506.937, "y"=177.78967, "z"=0.9839219}, "UV"={"u"=0.0, "v"=0.0}, "Colour"=12517256}, "Vertex 3"={"Position"={"x"=456.35504, "y"=174.77179, "z"=0.9835236}, "UV"={"u"=0.0, "v"=0.0}, "Colour"=12517256}, "Alpha"=0.0, "Alpha Blending Enabled"=FALSE, "Colour"=9091426}, {"Vertex 1"={"Position"={"x"=453.97424, "y"=135.72502, "z"=0.9837993}, "UV"={"u"=0.0, "v"=0.0}, "Colour"=12517256}, "Vertex 2"={"Position"={"x"=455.7062, "y"=153.40399, "z"=0.9835987}, "UV"={"u"=0.0, "v"=0.0}, "Colour"=12517256}, "Vertex 3"={"Position"={"x"=505.73492, "y"=156.89722, "z"=0.9839907}, "UV"={"u"=0.0, "v"=0.0}, "Colour"=12517256}, "Alpha"=0.0, "Alpha Blending Enabled"=FALSE, "Colour"=5402171}, {"Vertex 1"={"Position"={"x"=456.01822, "y"=198.56883, "z"=0.9835626}, "UV"={"u"=0.0, "v"=0.0}, "Colour"=12517256}, "Vertex 2"={"Position"={"x"=455.0632, "y"=223.28236, "z"=0.9836732}, "UV"={"u"=0.0, "v"=0.0}, "Colour"=12517256}, "Vertex 3"={"Position"={"x"=504.54324, "y"=225.08987, "z"=0.98405904}, "UV"={"u"=0.0, "v"=0.0}, "Colour"=12517256}, "Alpha"=0.0, "Alpha Blending Enabled"=FALSE, "Colour"=9816170}, {"Vertex 1"={"Position"={"x"=344.93683, "y"=223.28236, "z"=0.9836732}, "UV"={"u"=0.0, "v"=0.0}, "Colour"=12517256}, "Vertex 2"={"Position"={"x"=346.41867, "y"=248.47368, "z"=0.98384476}, "UV"={"u"=0.0, "v"=0.0}, "Colour"=12517256}, "Vertex 3"={"Position"={"x"=400.0, "y"=248.05318, "z"=0.98371255}, "UV"={"u"=0.0, "v"=0.0}, "Colour"=12517256}, "Alpha"=0.0, "Alpha Blending Enabled"=FALSE, "Colour"=10540915}, {"Vertex 1"={"Position"={"x"=344.93683, "y"=223.28236, "z"=0.9836732}, "UV"={"u"=0.0, "v"=0.0}, "Colour"=12517256}, "Vertex 2"={"Position"={"x"=343.98178, "y"=198.56883, "z"=0.9835626}, "UV"={"u"=0.0, "v"=0.0}, "Colour"=12517256}, "Vertex 3"={"Position"={"x"=293.68674, "y"=200.99902, "z"=0.98395765}, "UV"={"u"=0.0, "v"=0.0}, "Colour"=12517256}, "Alpha"=0.0, "Alpha Blending Enabled"=FALSE, "Colour"=9816170}, {"Vertex 1"={"Position"={"x"=343.64493, "y"=174.77179, "z"=0.9835236}, "UV"={"u"=0.0, "v"=0.0}, "Colour"=12517256}, "Vertex 2"={"Position"={"x"=344.29382, "y"=153.40399, "z"=0.9835987}, "UV"={"u"=0.0, "v"=0.0}, "Colour"=12517256}, "Vertex 3"={"Position"={"x"=294.26508, "y"=156.89722, "z"=0.9839907}, "UV"={"u"=0.0, "v"=0.0}, "Colour"=12517256}, "Alpha"=0.0, "Alpha Blending Enabled"=FALSE, "Colour"=7576403}, {"Vertex 1"={"Position"={"x"=400.0, "y"=222.63887, "z"=0.98353577}, "UV"={"u"=0.0, "v"=0.0}, "Colour"=12517256}, "Vertex 2"={"Position"={"x"=400.0, "y"=248.05318, "z"=0.98371255}, "UV"={"u"=0.0, "v"=0.0}, "Colour"=12517256}, "Vertex 3"={"Position"={"x"=453.58133, "y"=248.47368, "z"=0.98384476}, "UV"={"u"=0.0, "v"=0.0}, "Colour"=12517256}, "Alpha"=0.0, "Alpha Blending Enabled"=FALSE, "Colour"=10540915}, {"Vertex 1"={"Position"={"x"=455.7062, "y"=153.40399, "z"=0.9835987}, "UV"={"u"=0.0, "v"=0.0}, "Colour"=12517256}, "Vertex 2"={"Position"={"x"=453.97424, "y"=135.72502, "z"=0.9837993}, "UV"={"u"=0.0, "v"=0.0}, "Colour"=12517256}, "Vertex 3"={"Position"={"x"=400.0, "y"=134.37457, "z"=0.9836657}, "UV"={"u"=0.0, "v"=0.0}, "Colour"=12517256}, "Alpha"=0.0, "Alpha Blending Enabled"=FALSE, "Colour"=5599805}, {"Vertex 1"={"Position"={"x"=453.58133, "y"=248.47368, "z"=0.98384476}, "UV"={"u"=0.0, "v"=0.0}, "Colour"=12517256}, "Vertex 2"={"Position"={"x"=455.0632, "y"=223.28236, "z"=0.9836732}, "UV"={"u"=0.0, "v"=0.0}, "Colour"=12517256}, "Vertex 3"={"Position"={"x"=400.0, "y"=222.63887, "z"=0.98353577}, "UV"={"u"=0.0, "v"=0.0}, "Colour"=12517256}, "Alpha"=0.0, "Alpha Blending Enabled"=FALSE, "Colour"=10540915}, {"Vertex 1"={"Position"={"x"=455.7062, "y"=153.40399, "z"=0.9835987}, "UV"={"u"=0.0, "v"=0.0}, "Colour"=12517256}, "Vertex 2"={"Position"={"x"=456.35504, "y"=174.77179, "z"=0.9835236}, "UV"={"u"=0.0, "v"=0.0}, "Colour"=12517256}, "Vertex 3"={"Position"={"x"=506.937, "y"=177.78967, "z"=0.9839219}, "UV"={"u"=0.0, "v"=0.0}, "Colour"=12517256}, "Alpha"=0.0, "Alpha Blending Enabled"=FALSE, "Colour"=7576403}, {"Vertex 1"={"Position"={"x"=456.35504, "y"=174.77179, "z"=0.9835236}, "UV"={"u"=0.0, "v"=0.0}, "Colour"=12517256}, "Vertex 2"={"Position"={"x"=456.01822, "y"=198.56883, "z"=0.9835626}, "UV"={"u"=0.0, "v"=0.0}, "Colour"=12517256}, "Vertex 3"={"Position"={"x"=506.31323, "y"=200.99902, "z"=0.98395765}, "UV"={"u"=0.0, "v"=0.0}, "Colour"=12517256}, "Alpha"=0.0, "Alpha Blending Enabled"=FALSE, "Colour"=9091426}, {"Vertex 1"={"Position"={"x"=343.98178, "y"=198.56883, "z"=0.9835626}, "UV"={"u"=0.0, "v"=0.0}, "Colour"=12517256}, "Vertex 2"={"Position"={"x"=343.64493, "y"=174.77179, "z"=0.9835236}, "UV"={"u"=0.0, "v"=0.0}, "Colour"=12517256}, "Vertex 3"={"Position"={"x"=293.06296, "y"=177.78967, "z"=0.9839219}, "UV"={"u"=0.0, "v"=0.0}, "Colour"=12517256}, "Alpha"=0.0, "Alpha Blending Enabled"=FALSE, "Colour"=9091426}, {"Vertex 1"={"Position"={"x"=400.0, "y"=152.15985, "z"=0.9834591}, "UV"={"u"=0.0, "v"=0.0}, "Colour"=12517256}, "Vertex 2"={"Position"={"x"=400.0, "y"=134.37457, "z"=0.9836657}, "UV"={"u"=0.0, "v"=0.0}, "Colour"=12517256}, "Vertex 3"={"Position"={"x"=346.02576, "y"=135.72502, "z"=0.9837993}
